vi "Generate Audio Analyzer DVR.vi"(8 "Error In":errorcluster, 11 "Audio Analyzer In":refnum<class "Audio Analyzer.lvclass">) -> (0 "Error Out":errorcluster, 3 "Audio Analyzer Out":refnum<class "Audio Analyzer.lvclass">)   [LabVIEW 2019, in "Audio Analyzer.lvclass"]
uses:
  Audio Analyzer.lvclass
  Controls/Data.ctl
  Public/Controls/FPGA Reference.ctl
  Audio Analyzer.lvclass/Audio Analyzer.ctl
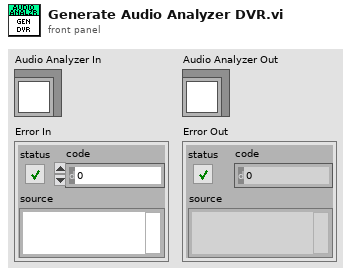
[diagram p1: front panel]
types:
  T1 = typedef "Audio Analyzer.lvclass/Data.ctl" = cluster{"Audio Spectrum Notifier":refnum<notifier>, "FPGA Reference":T2}
  T2 = typedef "Audio Analyzer.lvclass/FPGA Reference.ctl" = refnum<k20>
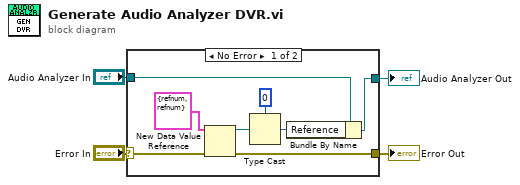
[diagram p0: block diagram]
diagram:
  n1 = case shown="No Error" "Error In" {
    selector: "Error In" -> [w12 w14]
    tunnel: "Audio Analyzer In" -> [w9 w13]
    tunnel: [w8 w13] -> w3
    tunnel: [w7 w14] -> w1
    frame No Error {
      n2 = New Data Value Reference(data value=T1 {"Audio Spectrum Notifier"=refnum, "FPGA Reference"=refnum} ("Data"), error in=w12) -> (data value reference=w11:refnum<data-value>, error out=w7:errorcluster)
      n3 = Type Cast(type=u64 0, x=w11) -> (*(type *) &x=w6:u64)
      n4 = Bundle By Name(cluster=w9, "Reference"=w6) -> (w8:refnum<class "Audio Analyzer.lvclass">)
    }
    frame Error {
    }
  }
  "Error Out" <- w1
  "Audio Analyzer Out" <- w3
